vi "RD_WR close.vi"(8 "error in":errorcluster, 11 "RD_WR param":T1) -> (0 "error out":errorcluster)   [LabVIEW 2021, in "ICPCON_Param.lvlib"]
uses:
  ICPCON_Param.lvlib
  ICPCON Param.ctl
  Eth timeouts.ctl
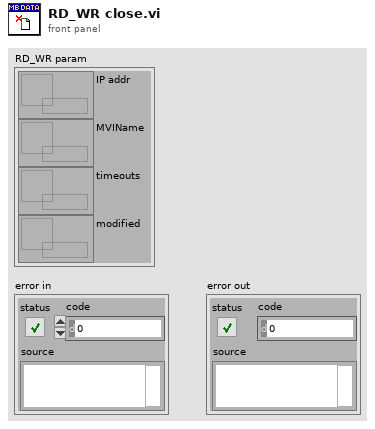
[diagram p1: front panel]
types:
  T1 = typedef "ICPCON_Param.lvlib/ICPCON Param.ctl" = cluster{"IP addr":refnum<data-value>, "MVIName":refnum<data-value>, "timeouts":refnum<data-value>, "modified":refnum<data-value>}
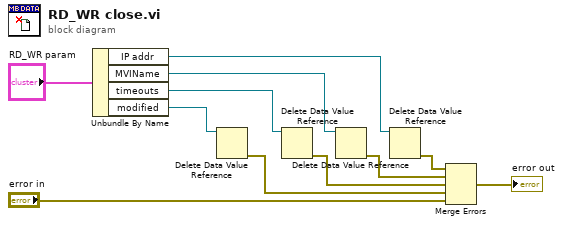
[diagram p0: block diagram]
diagram:
  n1 = Unbundle By Name("RD_WR param") -> ("IP addr"=w8:refnum<data-value>, "MVIName"=w9:refnum<data-value>, "timeouts"=w10:refnum<data-value>, "modified"=w3:refnum<data-value>)
  n2 = Delete Data Value Reference(data value reference=w3) -> (error out=w1:errorcluster)  [unwired: 1 in, 1 out]
  n3 = Delete Data Value Reference(data value reference=w10) -> (error out=w7:errorcluster)  [unwired: 1 in, 1 out]
  n4 = Delete Data Value Reference(data value reference=w9) -> (error out=w6:errorcluster)  [unwired: 1 in, 1 out]
  n5 = Delete Data Value Reference(data value reference=w8) -> (error out=w5:errorcluster)  [unwired: 1 in, 1 out]
  n6 = Merge Errors(w5, w6, w7, w1, "error in") -> (→"error out":errorcluster)
